vi "SubVI_Controle_velocidade_servo.vi"(8 "Link":i32, 9 "Posição Desejada":dbl, 10 "Posição":dbl, 11 "milliseconds to wait":u32) -> (2 "Duty Cycle":dbl(slide)=1.5 scale=0.025..0.125, 3 "Posição":dbl(knob)=1.5 scale=0.0..200.0)   [LabVIEW 2017]
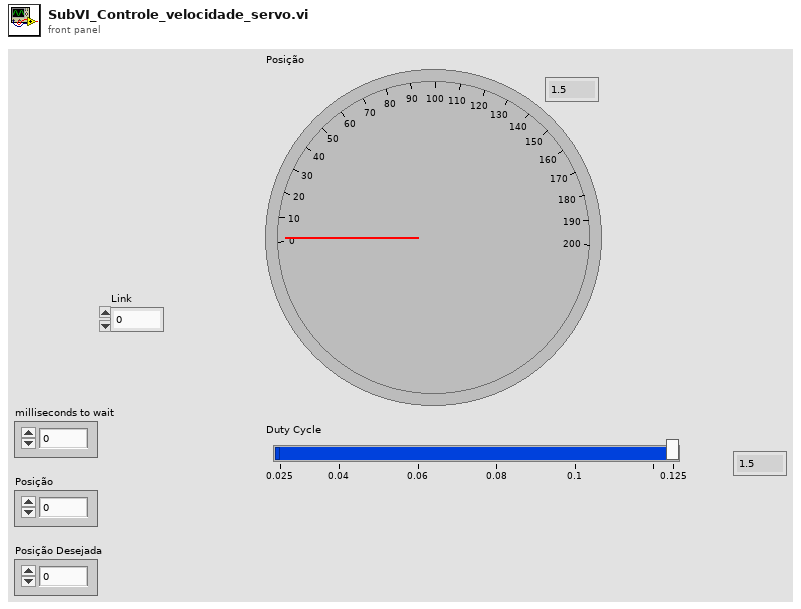
[diagram p1: front panel]
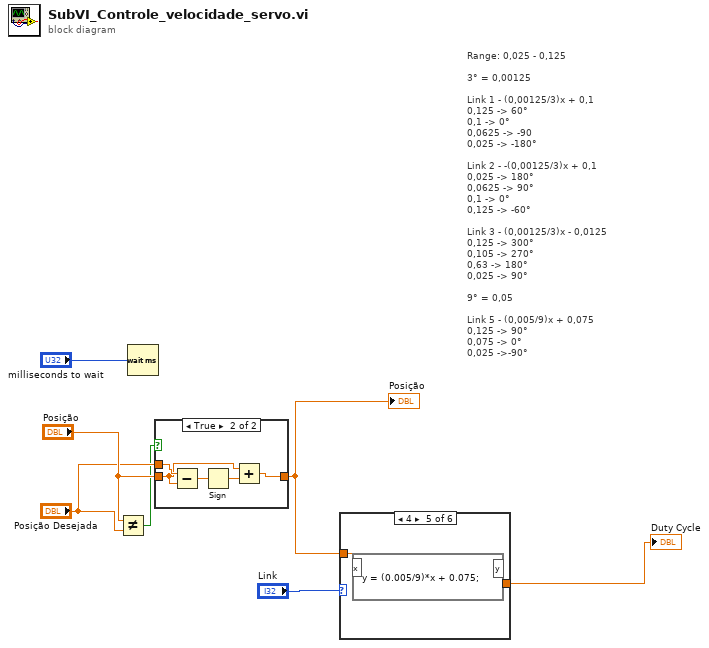
[diagram p0: block diagram]
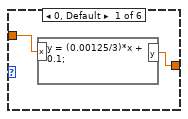
[diagram p2: hidden frame]
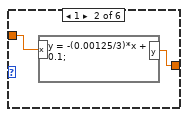
[diagram p3: hidden frame]
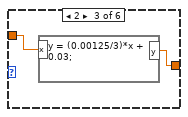
[diagram p4: hidden frame]
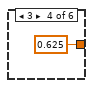
[diagram p5: hidden frame]
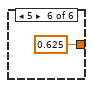
[diagram p6: hidden frame]
diagram:
  # "Range: 0,025 - 0,125\n\n3° = 0,00125\n\nLink 1 - (0,00125/3)x + 0,1\n0,125 -> 60°\n0,1 -> 0°\n0,0625 -> -90\n0,025 -> -180°\n\nLink 2 - -(0,00125/3)x + 0,1\n0,025 -> 180°\n0,0625 -> 90°\n0,1 -> 0°\n0,125 -> -60°\n\nLink 3 - (0,00125/3)x - 0,0125\n0,125 -> 300°\n0,105 -> 270° \n0,63 -> 180°\n0,025 -> 90°\n\n9° = 0,05\n\nLink 5 - (0,005/9)x + 0,075\n0,125 -> 90°\n0,075 -> 0°\n0,025 ->-90°"
  n1 = Not Equal?(x="Posição", y="Posição Desejada") -> (x != y?=w4:bool)
  n2 = Wait (ms)(milliseconds to wait="milliseconds to wait") -> ()  [unwired: 1 out]
  n3 = case shown="True" w4 {
    tunnel: "Posição Desejada" -> [_ w13]
    tunnel: "Posição" -> [w8 w11]
    tunnel: [w8 w10] -> w1
    frame False {
    }
    frame True {
      n4 = Subtract(x=w13, y=w11) -> (x-y=w12:dbl)
      n5 = Sign(1:w12) -> (0:w9:dbl)
      n6 = Add(x=w11, y=w9) -> (x+y=w10:dbl)
    }
  }
  "Posição" <- w1
  n7 = case shown="4" "Link" {
    tunnel: [w15 w16 w18 0.625 ("y") w21 0.625 ("y")] -> w2
    tunnel: w1 -> [w14 w17 w19 _ w22 _]
    frame 0, Default {
      n8 = formula code="y = (0.00125/3)*x + 0.1;"("x"=w14) -> ("y"=w15:dbl)
    }
    frame 1 {
      n9 = formula code="y = -(0.00125/3)*x + 0.1;"("x"=w17) -> ("y"=w16:dbl)
    }
    frame 2 {
      n10 = formula code="y = (0.00125/3)*x + 0.03;"("x"=w19) -> ("y"=w18:dbl)
    }
    frame 3 {
    }
    frame 4 {
      n11 = formula code="y = (0.005/9)*x + 0.075;"("x"=w22) -> ("y"=w21:dbl)
    }
    frame 5 {
    }
  }
  "Duty Cycle" <- w2
